vi "Find Distance.vi"(1 "Time (ms)":dbl, 2 "RPM":dbl) -> (0 "Distance":dbl)   [LabVIEW 2014]
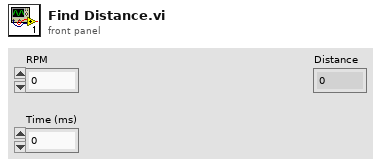
[diagram p1: front panel]
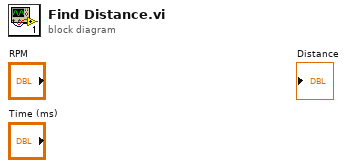
[diagram p0: block diagram]
diagram:
